vi "Close MeasurementLink Session.vi"(8 "error in":errorcluster, 9 "initialize and close session behavior":T1, 10 "session in":variant, 11 "session factory in":refnum<class "Abstract_Instrument.lvclass">) -> (0 "error out":errorcluster)   [LabVIEW 2020, in "Abstract_Instrument.lvclass"]
doc: "Closes the local session. If the session represents a remote session, <b>initialize and close session behavior</b> determines whether closing the local session closes the server session or detaches from the server session."
uses:
  Abstract_Instrument.lvclass
  <vilib>/MeasurementLink/MeasurementLink Instrument/ISession Factory/Initialize and Close Session Behavior.ctl
  <vilib>/MeasurementLink/MeasurementLink Instrument/ISession Factory/ISession Factory.lvclass
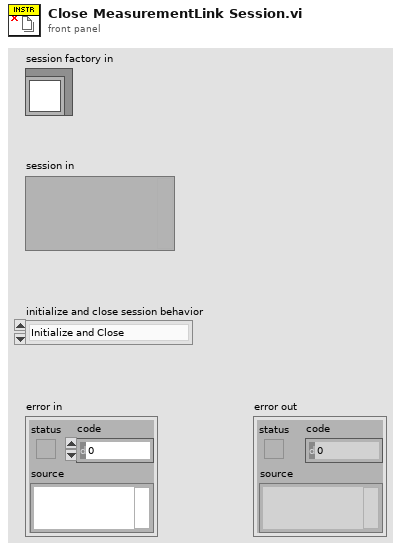
[diagram p1: front panel]
types:
  T1 = typedef "MeasurementLink Instrument.lvlib/ISession Factory.lvclass/Initialize and Close Session Behavior.ctl" = enum16{"Initialize and Close", "Attach and Detach", "Initialize and Detach", "Attach and Close"}
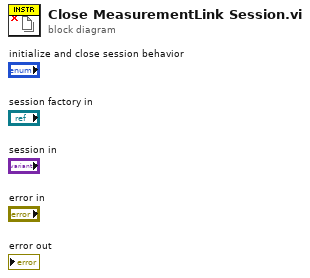
[diagram p0: block diagram]
diagram:
